vi "IV_BMT_K2410.vi"() -> ()   [LabVIEW 2010]
uses:
  <vilib>/Utility/file.llb/Write To Spreadsheet File (DBL).vi
panel:
  in  "Write Module ID Folder":string="Module_Digital<#>"
  out "error out":errorcluster
  out "I/V Graph":cluster{"trace":dbl[], "trace":dbl[]}(graph)={"trace"=[0.0, -1.178974, -2.994318, -5.35106, -8.158611, -11.34021, -14.83203, -18.58115, -22.54368, -26.68321, -30.96954, -35.37762, -39.88668, -44.47951, -49.1418, -53.8617, -58.62939, -63.43671, -68.2769, -73.14436, -78.03443, -82.94325, -87.86763, -92.80492, -97.75289, -102.7097, -107.674, -112.6443, -117.6197, -122.5993, -127.5823, -132.5683, -137.5566, -142.547, -147.539, -152.5323, -157.5268, -162.5222, -167.5184, -172.5153, -177.5127, -182.5105, -187.5087, -192.5072, -197.506, -202.505, -207.5041, -212.5034, -217.5029, -222.5024, -227.502, -232.5016, -237.5014, -242.5011, -247.5009, -252.5008, -257.5006, -262.5005, -267.5005, -272.5004, -277.5003], "trace"=[-1.94794e-08, -1.524239e-07, -2.643114e-07, -3.584467e-07, -4.404427e-07, -5.105356e-07, -5.737728e-07, -6.260196e-07, -6.734326e-07, -7.130487e-07, -7.512526e-07, -7.73741e-07, -7.841596e-07, -7.890017e-07, -7.941103e-07, -7.984052e-07, -8.033478e-07, -8.094917e-07, -8.145474e-07, -8.192927e-07, -8.25183e-07, -8.304166e-07, -8.365462e-07, -8.418278e-07, -8.444512e-07, -8.49288e-07, -8.51472e-07, -8.548865e-07, -8.583729e-07, -8.611872e-07, -8.660323e-07, -8.687162e-07, -8.726046e-07, -8.762418e-07, -8.790543e-07, -8.8295e-07, -8.83947e-07, -8.881656e-07, -8.920854e-07, -8.951716e-07, -8.982292e-07, -9.007702e-07, -9.054235e-07, -9.087858e-07, -9.124051e-07, -9.162425e-07, -9.189004e-07, -9.232807e-07, -9.257591e-07, -9.299052e-07, -9.335167e-07, -9.382692e-07, -9.424057e-07, -9.466199e-07, -9.515715e-07, -9.559809e-07, -9.612983e-07, -9.658505e-07, -9.703045e-07, -9.750671e-07, -9.800574e-07]}
  in  "error in":errorcluster
  in  "measurement":string(combo)="IV"
  in  "Filename":path=path "D:/pixelsensor/Module_Digital9/IV_Module_Digital.txt"
  in  "abort measurement":bool
  in  "Start voltage Bias":dbl
  in  "Compliance [A]":dbl=3e-05 format="%.1p"
  in  "Save in File":bool=TRUE
  in  "Wait [ms]":dbl=3000.0
  in  "Stepsize bias [V]":dbl=-5.0 format="%.1f"
  in  "Voltage Max [V]":dbl=-300.0
  # "IV Measurement"
  # "Module Production 2014"
  # "BARE MODULE TEST"
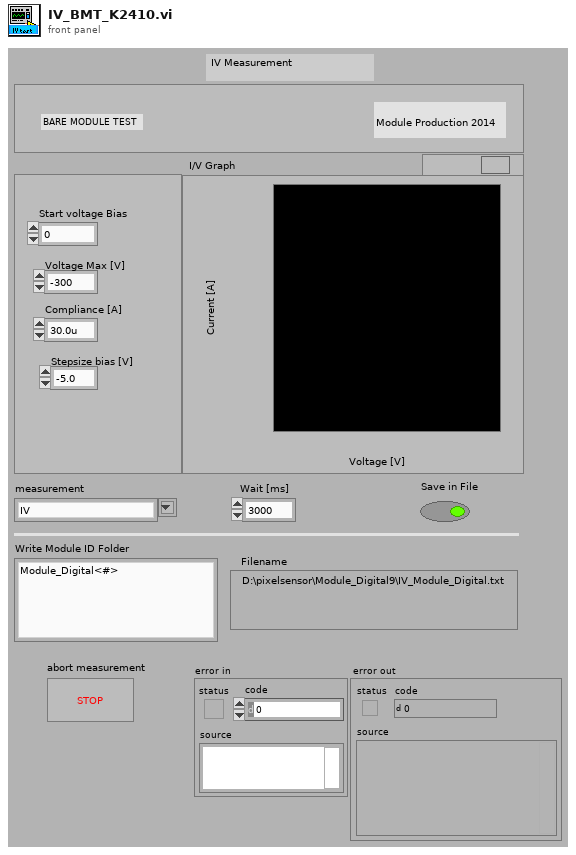
[diagram p1: front panel]
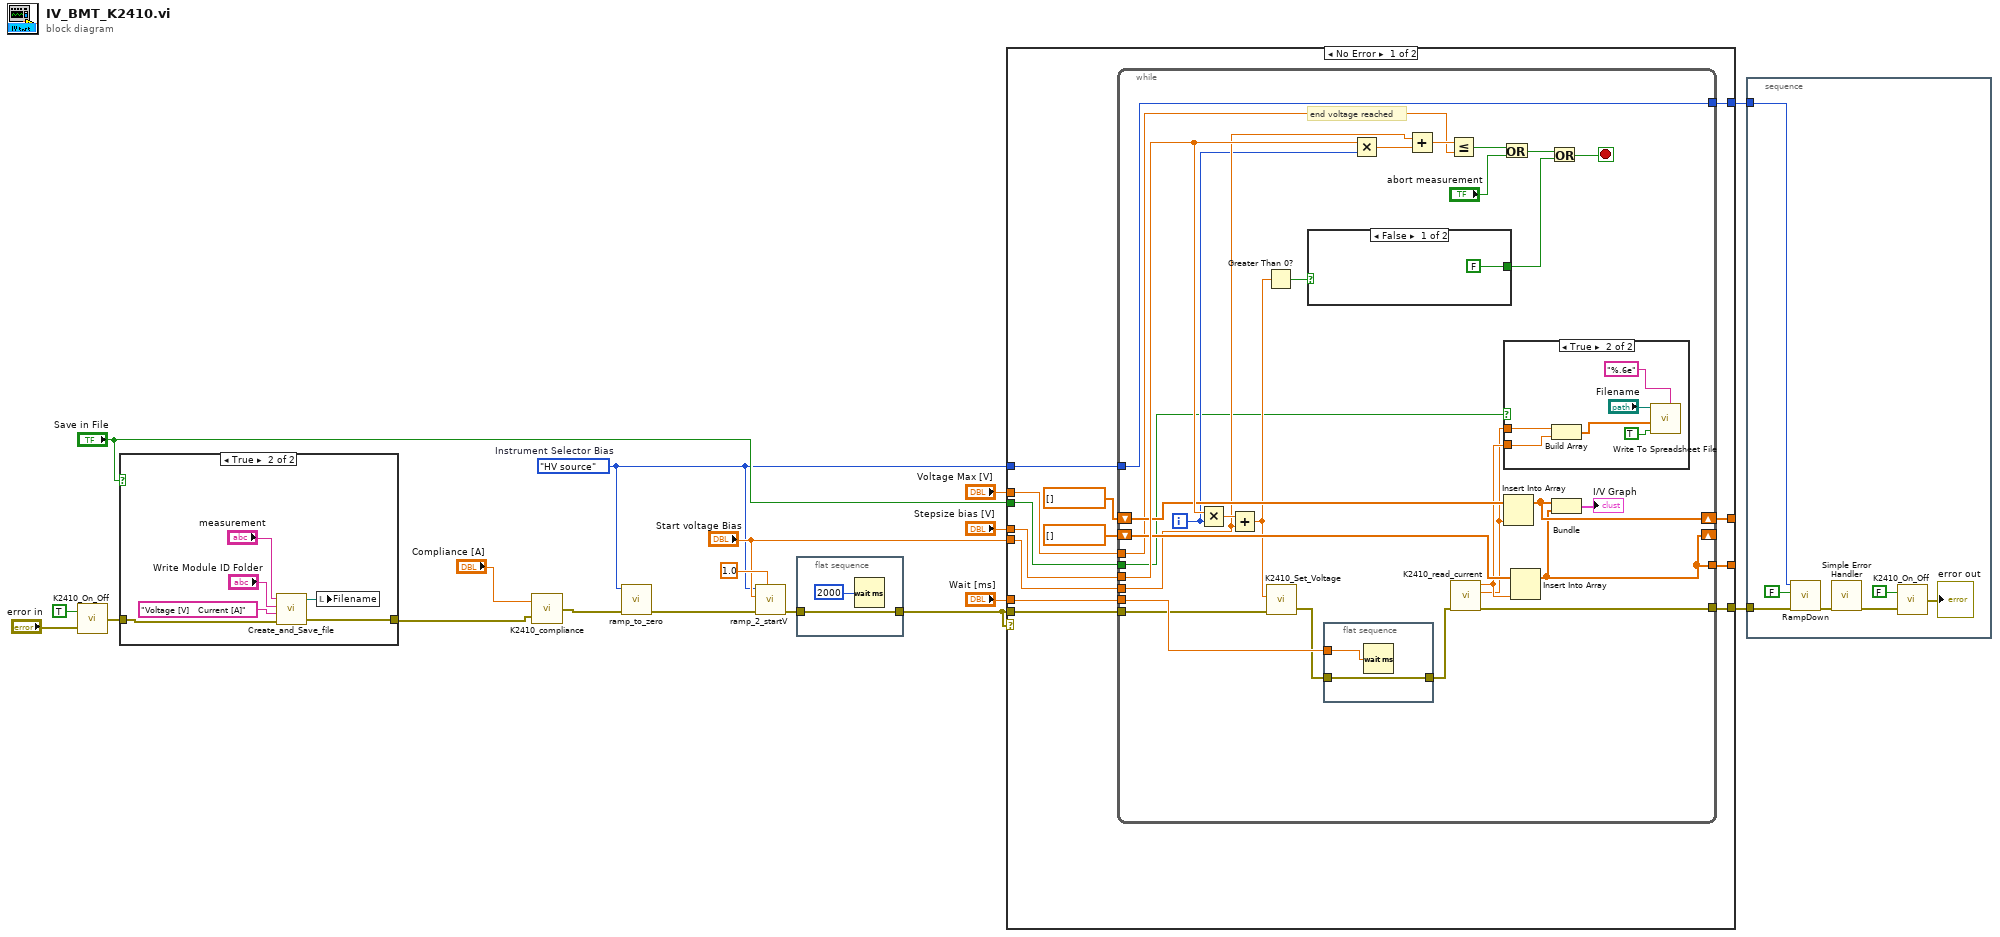
[diagram p0: block diagram]
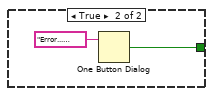
[diagram p3: hidden frame]
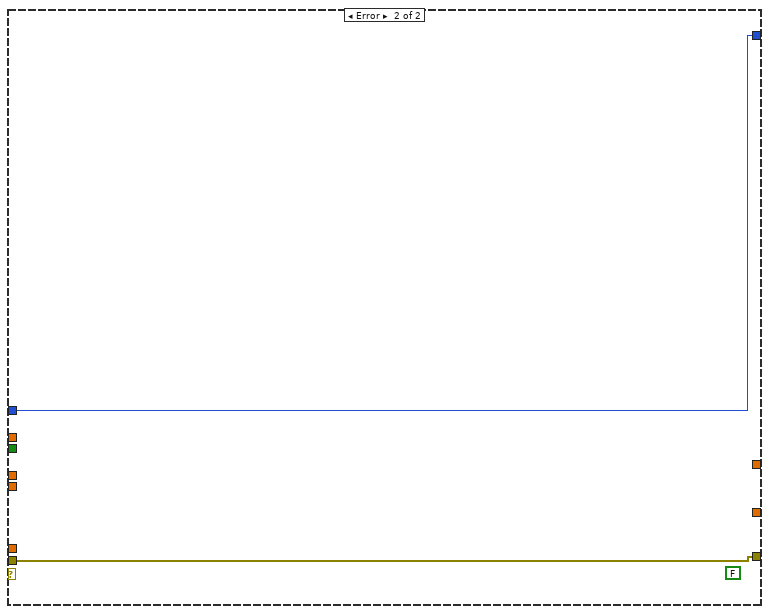
[diagram p5: hidden frame]
diagram:
  w4 = enum16{"HV source", " V source"}."HV source"  # Instrument Selector Bias
  n1 = call "K2410_On_Off.vi"("error in"="error in", "On/Off"=TRUE) -> ("error out"=w10:errorcluster)
  n2 = case shown="True" "Save in File" {
    tunnel: [w19 w23] -> w2
    tunnel: w10 -> [w19 w21]
    frame False {
    }
    frame True {
      n3 = call "Create_and_Save_file.vi"("measurement"="measurement", "OBJECT_ID (and relative Filepath)"="Write Module ID Folder", "Header1"="Voltage [V]   Current [A]", "error in"=w21) -> ("filename"=w22:path, "error out"=w23:errorcluster)  [unwired: 2 in]
      n4 = local write "Filename"(w22) -> ()
    }
  }
  n5 = call "K2410_compliance.vi"("error in"=w2, "Compliance [A]"="Compliance [A]") -> ("error out"=w1:errorcluster)
  n6 = call "ramp_to_zero.vi"("error in"=w1, "Instrument Selector"=w4) -> ("error out"=w8:errorcluster)  [unwired: 9 in]
  n7 = call "ramp_2_startV.vi"("Ramp_rate(0.5 -10V)"=1.0 ("Ramp_rate(0.5 -10V) Bias"), "error in"=w8, "Start voltage"="Start voltage Bias", "Instrument Selector"=w4) -> ("error out"=w7:errorcluster)  [unwired: 7 in]
  n8 = flat-sequence {
    tunnel: w7 -> [w27]
    tunnel: [w27] -> w13
    frame #0 {
      n9 = Wait (ms)(milliseconds to wait=u32 2000) -> ()  [unwired: 1 out]
    }
  }
  n10 = case shown="No Error" w13 {
    tunnel: "Stepsize bias [V]" -> [w40 _]
    tunnel: [w28 w81] -> w14
    tunnel: "Voltage Max [V]" -> [w37 _]
    tunnel: "Save in File" -> [w36 _]
    tunnel: [w35 _] -> _
    tunnel: [w34 _] -> _
    tunnel: "Start voltage Bias" -> [w33 _]
    tunnel: w13 -> [w32 w81]
    tunnel: "Wait [ms]" -> [w31 _]
    tunnel: [w30 w80] -> w6
    tunnel: w4 -> [w29 w80]
    frame No Error {
      n11 = while {
        tunnel: w36 -> [w44]
        tunnel: w37 -> [w49]
        shift-left: dbl[] [] -> [w63]
        shift-right: [w61] -> w35
        shift-left: dbl[] [] -> [w62]
        shift-right: [w52] -> _
        tunnel: w40 -> [w68]
        tunnel: [w52] -> w34
        tunnel: w33 -> [w55]
        tunnel: w32 -> [w45]
        tunnel: w31 -> [w64]
        tunnel: [w54] -> w30
        tunnel: w29 -> [w54]
        tunnel: [w43] -> w28
        i -> [w48]
        stop <- w50 stop-if-true
        # "end voltage reached"
        n12 = Multiply(x=w68, y=w48) -> (x*y=w67:dbl)
        n13 = Add(x=w67, y=w55) -> (x+y=w53:dbl)
        n14 = Greater Than 0?(x=w53) -> (x > 0?=w47:bool)
        n15 = call "K2410_Set_Voltage.vi"("error in"=w45, "VoltageLevel"=w53) -> ("error out"=w42:errorcluster)  [unwired: 3 in]
        n16 = case shown="False" w47 {
          tunnel: [FALSE w71] -> w46
          frame False {
          }
          frame True {
            n17 = One Button Dialog(message="Error...positive bias") -> (true=w71:bool)  [unwired: 1 in]
          }
        }
        n18 = flat-sequence {
          tunnel: [w73] -> w41
          tunnel: w42 -> [w73]
          tunnel: w64 -> [w72]
          frame #0 {
            n19 = Wait (ms)(milliseconds to wait=w72) -> ()  [unwired: 1 out]
          }
        }
        n20 = Multiply(x=w68, y=w48) -> (x*y=w66:dbl)
        n21 = Add(x=w55, y=w66) -> (x+y=w59:dbl)
        n22 = Less Or Equal?(x=w59, y=w49) -> (x <= y?=w56:bool)
        n23 = call "K2410_read_current.vi"("error in"=w41) -> ("error out"=w43:errorcluster, "voltage [V]"=w57:dbl, "current [A]"=w60:dbl)  [unwired: 5 in, 1 out]
        n24 = Or(x=w56, y="abort measurement") -> (x .or. y?=w51:bool)
        n25 = case shown="True" w44 {
          tunnel: w60 -> [_ w75]
          tunnel: w57 -> [_ w74]
          frame False {
          }
          frame True {
            n26 = Build Array(w74, w75) -> (w76:dbl[])
            n27 = call-poly <vilib>:"Write To Spreadsheet File.vi"("format (%.3f)"="%.6e", "append to file? (new file:F)"=TRUE, "1D data"=w76, "file path (dialog if empty)"="Filename") -> ()  [unwired: 4 in, 1 out]
          }
        }
        n28 = Insert Into Array(array=w63, new element=w57) -> (w61:dbl[])  [unwired: 1 in]
        n29 = Insert Into Array(array=w62, new element=w60) -> (w52:dbl[])  [unwired: 1 in]
        n30 = Or(x=w51, y=w46) -> (x .or. y?=w50:bool)
        n31 = Bundle(w61, w52) -> (→"I/V Graph":cluster{dbl[], dbl[]})  [unwired: 1 in]
      }
    }
    frame Error {
      (unwired) FALSE ("compliance")
    }
  }
  n32 = stacked-sequence {
    tunnel: w14 -> [w86]
    tunnel: w6 -> [w83]
    frame #0 {
      n33 = call "RampDown.vi"("error in"=w86, "On/Off"=FALSE, "Instrument Selector"=w83) -> ("error out"=w87:errorcluster)  [unwired: 6 in]
      n34 = call <vilib>:"Simple Error Handler.vi"("error in (no error)"=w87) -> ("error out"=w85:errorcluster)  [unwired: 4 in, 4 out]
      n35 = call "K2410_On_Off.vi"("error in"=w85, "On/Off"=FALSE) -> ("error out"=→"error out":errorcluster)
    }
  }
